vi "Constructor.vi"(8 "error in (no error)":errorcluster, 11 "Facade in":refnum<class "Facade.lvclass">) -> (0 "error out":errorcluster, 3 "Facade out":refnum<class "Facade.lvclass">)   [LabVIEW 2013, in "Facade.lvclass"]
uses:
  Facade.lvclass
  CDPlayer.lvclass/CDPlayer.lvclass
  DVDPlayer.lvclass/DVDPlayer.lvclass
  Tuner.lvclass/Tuner.lvclass
  Projector.lvclass/Projector.lvclass
  Amplifer.lvclass/Amplifer.lvclass
  RoomLight.lvclass/RoomLight.lvclass
  Facade.lvclass/Facade.ctl
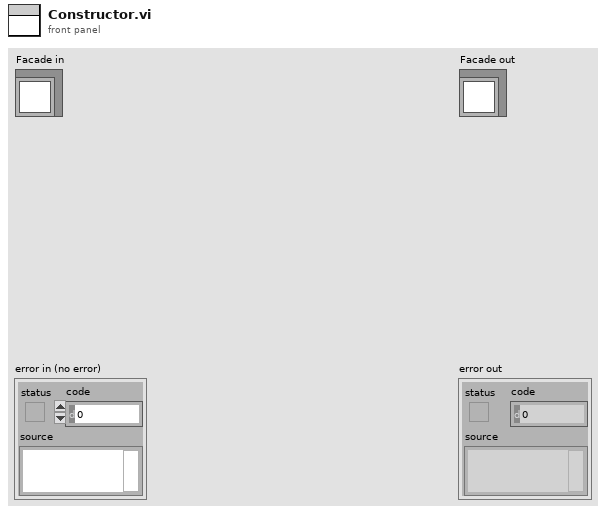
[diagram p1: front panel]
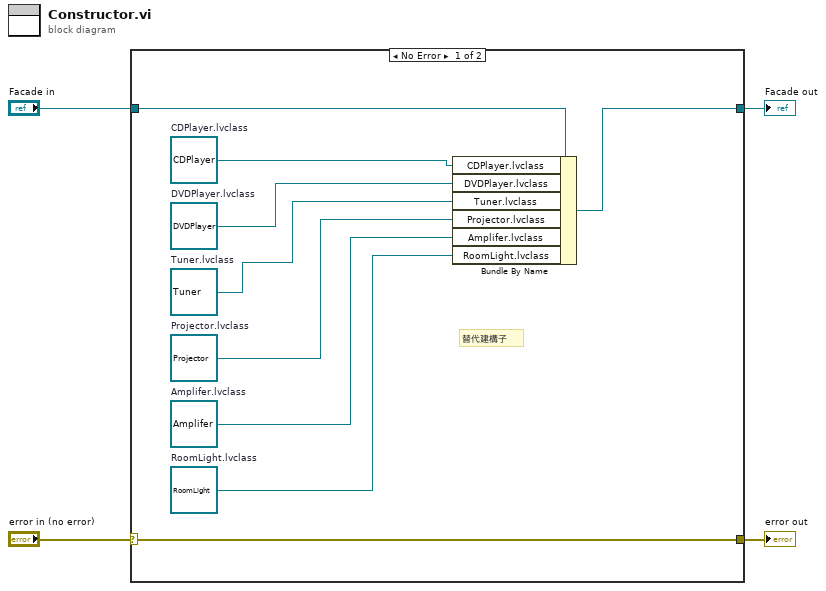
[diagram p0: block diagram]
diagram:
  n1 = case shown="No Error" "error in (no error)" {
    selector: "error in (no error)" -> [w13 w15]
    tunnel: [w13 w15] -> w3
    tunnel: [w5 w14] -> w1
    tunnel: "Facade in" -> [w6 w14]
    frame No Error {
      w7 = refnum<class "RoomLight.lvclass"> refnum  # RoomLight.lvclass
      w8 = refnum<class "Amplifer.lvclass"> refnum  # Amplifer.lvclass
      w9 = refnum<class "Projector.lvclass"> refnum  # Projector.lvclass
      w10 = refnum<class "Tuner.lvclass"> refnum  # Tuner.lvclass
      w11 = refnum<class "DVDPlayer.lvclass"> refnum  # DVDPlayer.lvclass
      w12 = refnum<class "CDPlayer.lvclass"> refnum  # CDPlayer.lvclass
      # "替代建構子"
      n2 = Bundle By Name(cluster=w6, "CDPlayer.lvclass"=w12, "DVDPlayer.lvclass"=w11, "Tuner.lvclass"=w10, "Projector.lvclass"=w9, "Amplifer.lvclass"=w8, "RoomLight.lvclass"=w7) -> (w5:refnum<class "Facade.lvclass">)
    }
    frame Error {
    }
  }
  "error out" <- w3
  "Facade out" <- w1
